vi "PD500 - Breaker AUX & Shunt Trip.vi"(8 "error in (no error)":errorcluster, 10 "Message IN":string) -> (0 "error out":errorcluster, 1 "Result (bool)":bool, 2 "Message OUT":string)   [LabVIEW 2022 SP3]
uses:
  <vilib>/DAQmx/write.llb/DAQmx Write (Digital Bool 1Line 1Point).vi
  <vilib>/DAQmx/read.llb/DAQmx Read (Digital 1D Bool NChan 1Samp 1Line).vi
  <vilib>/DAQmx/miscellaneous.llb/DAQmx Fill In Error Info.vi
panel:
  in  "bypass":bool
  in  "stop":bool
  out "Expected Breaker AUX state":bool[](array[boolean])
  out "Instructional Message":string
  in  "OK Button":bool
  out "Actual Breaker AUX state":bool[](array[boolean])
  out "Result (color)":u32(colorbox)
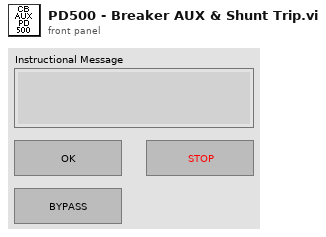
[diagram p1: front panel]
types:
  T1 = cluster{"Expected AUX State":bool[], "Inst. Message":string, "Shunt Trip":bool}[]
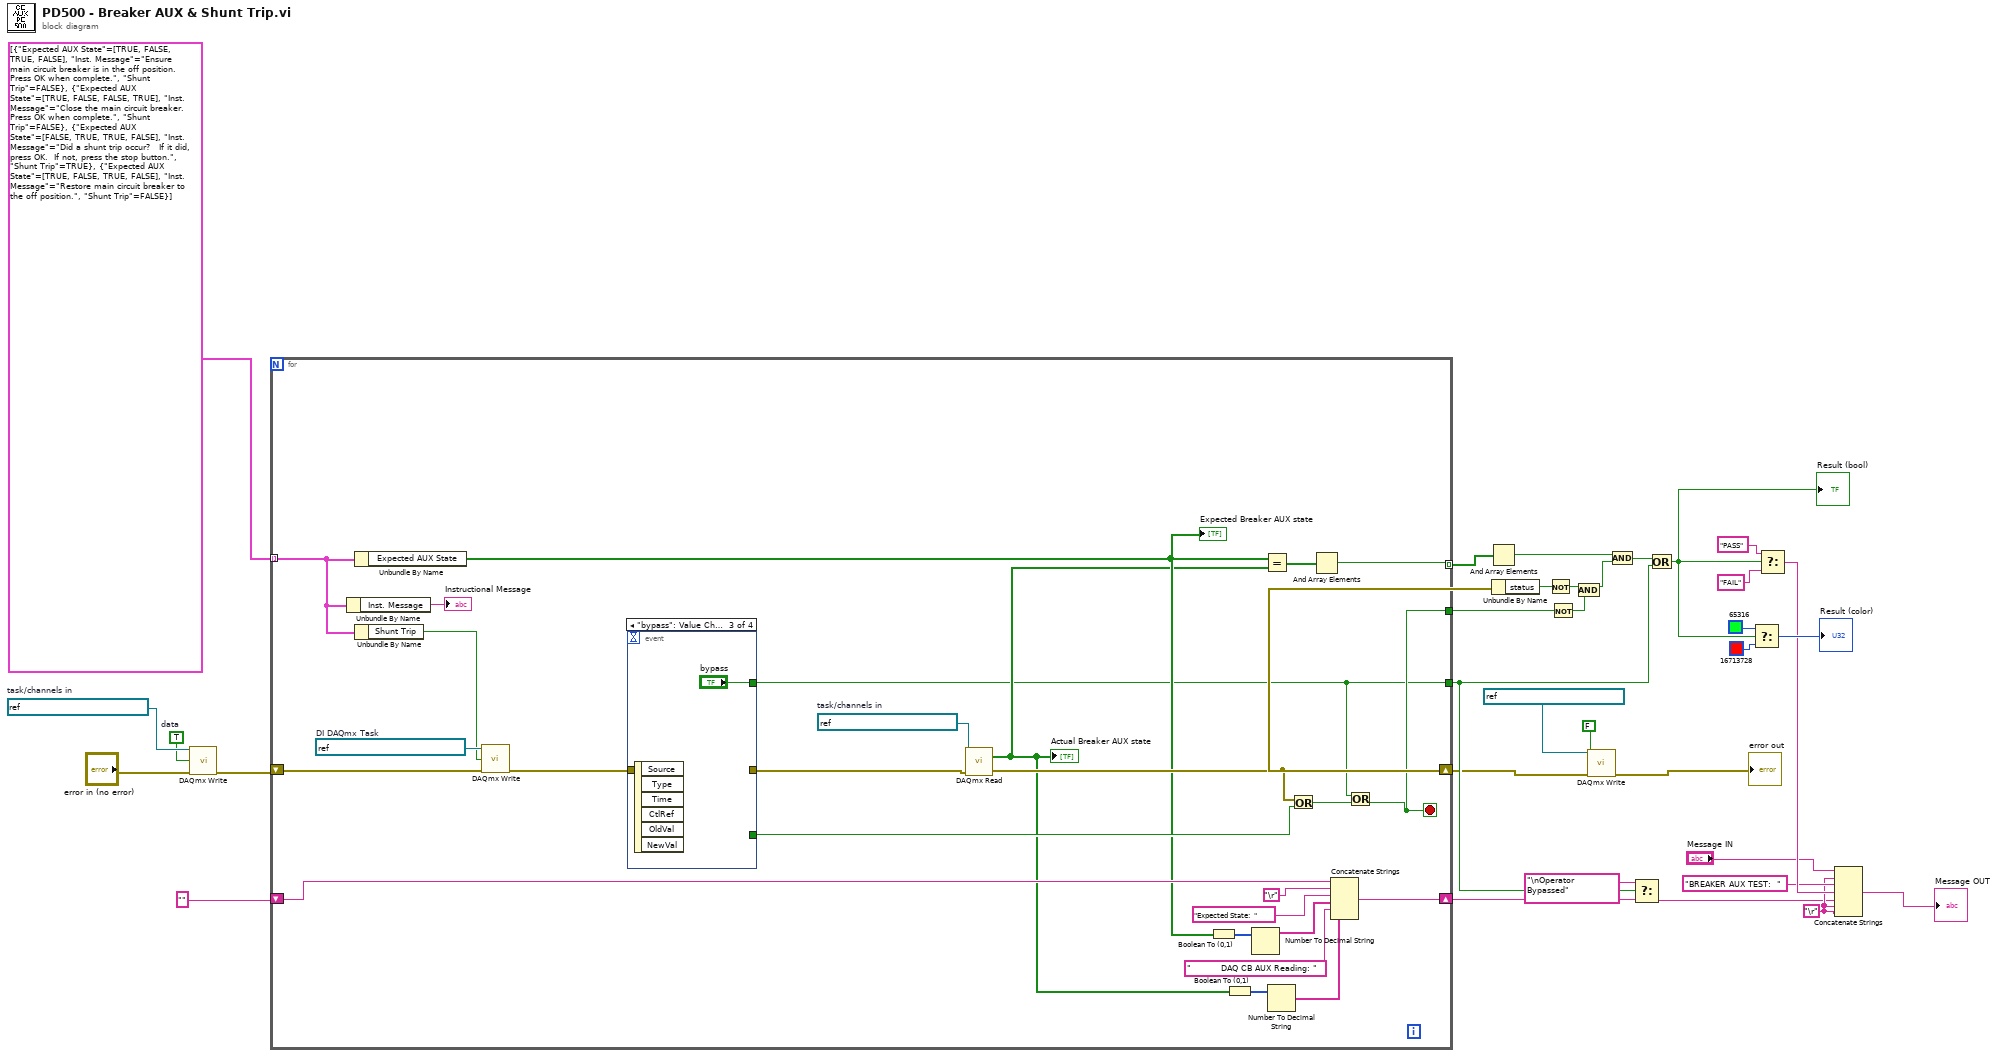
[diagram p0: block diagram]
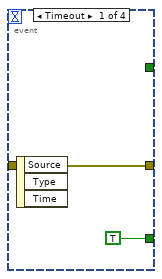
[diagram p2: hidden frame]
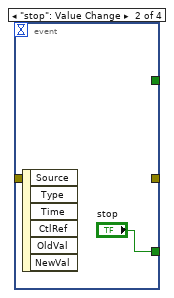
[diagram p3: hidden frame]
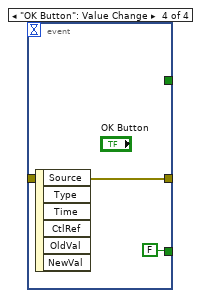
[diagram p4: hidden frame]
diagram:
  w16 = TRUE  # data
  w17 = refnum<k21> "FTS2_ProgrammingRelay"  # task/channels in
  w20 = "\r"
  n1 = call-poly <vilib>:"DAQmx Write.vi"("task/channels in"=w17, "data"=w16, "error in"="error in (no error)") -> ("error out"=w14:errorcluster)  [unwired: 10 in, 2 out]
  n2 = for {
    shift-right: [w41] -> w3
    shift-left: w14 -> [w47]
    tunnel: [w39] -> w33 mode=indexing
    shift-right: [w51] -> w7
    shift-left: "" -> [w50]
    tunnel: T1 [{"Expected AUX State"=[TRUE, FALSE, TRUE, FALSE], "Inst. Message"="Ensure main circuit breaker is in the off position.  Press OK when complete.", "Shunt Trip"=FALSE}, {"Expected AUX State"=[TRUE, FALSE, FALSE, TRUE], "Inst. Message"="Close the main circuit breaker.  Press OK when complete.", "Shunt Trip"=FALSE}, {"Expected AUX State"=[FALSE, TRUE, TRUE, FALSE], "Inst. Message"="Did a shunt trip occur?   If it did, press OK.  If not, press the stop button.", "Shunt Trip"=TRUE}, {"Expected AUX State"=[TRUE, FALSE, TRUE, FALSE], "Inst. Message"="Restore main circuit breaker to the off position.", "Shunt Trip"=FALSE}] -> [w42] mode=indexing
    tunnel: [w35] -> w11
    tunnel: [w34] -> w6
    stop <- w35 stop-if-true
    w48 = refnum<k21> "FTS2_PD500_BreakerAUX"  # task/channels in
    w59 = refnum<k21> "FTS2_PD500_MainACShunt"  # DI DAQmx Task
    n3 = Unbundle By Name(w42) -> ("Inst. Message"=→"Instructional Message":string)
    n4 = Unbundle By Name(w42) -> ("Expected AUX State"=w37:bool[])
    "Expected Breaker AUX state" <- w37
    n5 = Unbundle By Name(w42) -> ("Shunt Trip"=w43:bool)
    n6 = call-poly <vilib>:"DAQmx Write.vi"("task/channels in"=w59, "data"=w43, "error in"=w47) -> ("error out"=w46:errorcluster)  [unwired: 10 in, 2 out]
    n7 = event shown="[2] \"bypass\": Value Change" {
      selector: _ -> [_ _ _ _]
      dyn-events: _ -> [_ _ _ _]
      timeout: _ -> [_ _ _ _]
      tunnel: w46 -> [w61 _ _ w65]
      tunnel: [w61 _ _ w65] -> w45
      tunnel: [TRUE "stop" _ FALSE] -> w40
      tunnel: [_ _ "bypass" _] -> w34
      event Timeout {
        n8 = event-data() -> ()  [unwired: 1 in, 3 out]
      }
      event "stop": Value Change {
        n9 = event-data() -> ()  [unwired: 1 in, 6 out]
      }
      event "bypass": Value Change {
        n10 = event-data() -> ()  [unwired: 1 in, 6 out]
      }
      event "OK Button": Value Change {
        n11 = event-data() -> ()  [unwired: 1 in, 6 out]
      }
    }
    n12 = call-poly <vilib>:"DAQmx Read.vi"("task/channels in"=w48, "error in"=w45) -> ("data"=w36:bool[], "error out"=w41:errorcluster)  [unwired: 11 in, 1 out]
    "Actual Breaker AUX state" <- w36
    n13 = Boolean To (0,1)(Boolean=w37) -> (0, 1=w53:i16[])
    n14 = Boolean To (0,1)(Boolean=w36) -> (0, 1=w52:i16[])
    n15 = Number To Decimal String(number=w53) -> (decimal integer string=w56:string[])  [unwired: 1 in]
    n16 = Equal?(x=w37, y=w36) -> (x = y?=w49:bool[])
    n17 = Number To Decimal String(number=w52) -> (decimal integer string=w58:string[])  [unwired: 1 in]
    n18 = Or(x=w41, y=w40) -> (x .or. y?=w38:bool)
    n19 = And Array Elements(Boolean array=w49) -> (logical AND=w39:bool)
    n20 = Concatenate Strings(w50, "\r", "Expected State:  ", w56, "          DAQ CB AUX Reading: ", w58) -> (w51:string)
    n21 = Or(x=w34, y=w38) -> (x .or. y?=w35:bool)
  }
  n22 = And Array Elements(Boolean array=w33) -> (logical AND=w25:bool)
  n23 = Unbundle By Name(w3) -> ("status"=w27:bool)
  n24 = Not(x=w27) -> (.not. x?=w26:bool)
  n25 = Not(x=w11) -> (.not. x?=w12:bool)
  n26 = And(x=w26, y=w12) -> (x .and. y?=w13:bool)
  n27 = call-poly <vilib>:"DAQmx Write.vi"("task/channels in"=refnum<k21> "FTS2_ProgrammingRelay", "data"=FALSE, "error in"=w3) -> ("error out"=→"error out":errorcluster)  [unwired: 10 in, 2 out]
  n28 = And(x=w25, y=w13) -> (x .and. y?=w9:bool)
  n29 = Select(t="\nOperator Bypassed", s=w6, f=w7) -> (s? t:f=w8:string)
  n30 = Or(x=w9, y=w6) -> (x .or. y?=w10:bool)
  "Result (bool)" <- w10
  n31 = Select(t=u32 65316 ("Result (color)"), s=w10, f=u32 16713728 ("Result (color)")) -> (s? t:f=→"Result (color)":u32)
  n32 = Select(t="PASS", s=w10, f="FAIL") -> (s? t:f=w23:string)
  n33 = Concatenate Strings("Message IN", w20, "BREAKER AUX TEST:  ", w23, w8, w20, w20) -> (→"Message OUT":string)
